vi "On Change Camera Source.vi"(8 "error in (no error)":errorcluster, 10 "Selection":i32, 11 "App in":refnum<class "App.lvclass">) -> (0 "error out":errorcluster, 3 "App out":refnum<class "App.lvclass">)   [LabVIEW 2020, in "AR Example.lvlib" / "App.lvclass"]
uses:
  App.lvclass
  App.lvclass/App.ctl
  UI/UI.lvclass
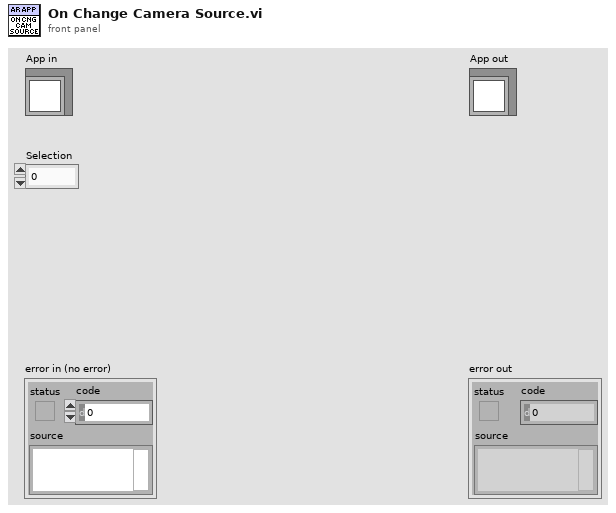
[diagram p1: front panel]
types:
  T1 = typedef "g_ar_toolkit.capture.lvlib/CameraManager.lvclass/Device Enumeration.ctl" = cluster{"Name":string, "Streams":set{T2}}
  T2 = typedef "g_ar_toolkit.capture.lvlib/CameraManager.lvclass/Stream Parameters.ctl" = cluster{"Width":u16, "Height":u16, "FPS":u8}
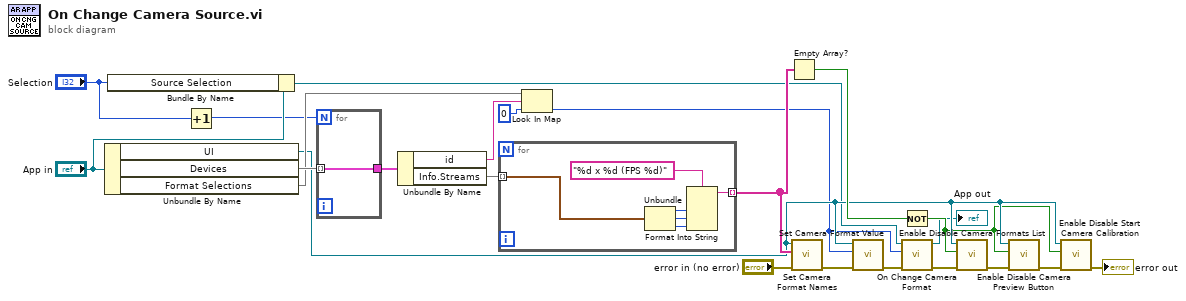
[diagram p0: block diagram]
diagram:
  n1 = Unbundle By Name("App in") -> ("UI"=w10:refnum<class "UI.lvclass">, "Devices"=w22:map{string, T1}, "Format Selections"=w18:map{string, i32})
  n2 = Bundle By Name(cluster="App in", "Source Selection"="Selection") -> (w5:refnum<class "App.lvclass">)
  n3 = Increment(x="Selection") -> (x+1=w1:i32)
  n4 = for {
    N: w1 -> [_]
    tunnel: w22 -> [w24] mode=indexing
    tunnel: [w24] -> w21
  }
  n5 = Unbundle By Name(w21) -> ("id"=w16:string, "Info.Streams"=w20:set{T2})
  n6 = for {
    tunnel: w20 -> [w30] mode=indexing
    tunnel: [w26] -> w14 mode=indexing
    n7 = Unbundle(w30) -> ("Width"=w29:u16, "Height"=w28:u16, "FPS"=w27:u8)
    n8 = Format Into String(format string="%d x %d (FPS %d)", w29, w28, w27) -> (resulting string=w26:string)  [unwired: 2 in, 1 out]
  }
  n9 = Look In Map(map=w18, key=w16, default value=0) -> (value=w6:i32)  [unwired: 1 out]
  n10 = Empty Array?(array=w14) -> (empty?=w13:bool)
  n11 = call-dynamic "Set Camera Format Names.vi"("error in (no error)"="error in (no error)", "Names"=w14, "UI in"=w10) -> ("error out"=w15:errorcluster)  [unwired: 8 in]
  n12 = call-dynamic "Set Camera Format Value.vi"("error in (no error)"=w15, "Value"=w6, "UI in"=w10) -> ("error out"=w7:errorcluster)  [unwired: 8 in]
  n13 = Not(x=w13) -> (.not. x?=w9:bool)
  n14 = call "On Change Camera Format.vi"("error in (no error)"=w7, "Selection"=w6, "App in"=w5) -> ("error out"=w3:errorcluster, "App out"=→"App out":refnum<class "App.lvclass">)  [unwired: 7 in]
  n15 = call-dynamic "Enable Disable Camera Formats List.vi"("error in (no error)"=w3, "Enable?"=w9, "UI in"=w10) -> ("error out"=w12:errorcluster)  [unwired: 8 in]
  n16 = call-dynamic "Enable Disable Camera Preview Button.vi"("error in (no error)"=w12, "Enable?"=w9, "UI in"=w10) -> ("error out"=w11:errorcluster)  [unwired: 8 in]
  n17 = call-dynamic "Enable Disable Start Camera Calibration.vi"("error in (no error)"=w11, "Enable?"=w9, "UI in"=w10) -> ("error out"=→"error out":errorcluster)  [unwired: 8 in]
